vi "onDestroy.vi"(8 "error in (no error)":errorcluster, 11 "Client in":refnum<class "Client.lvclass">) -> (0 "error out":errorcluster, 3 "Client out":refnum<class "Client.lvclass">)   [LabVIEW 2013, in "MQTT Client.lvlib" / "Client.lvclass"]
uses:
  Client.lvclass
  MQTT_Base/Base Class/MQTT_Base.lvclass
  Client.lvclass/Client.ctl
  MQTT_Base/Session/Session.lvclass
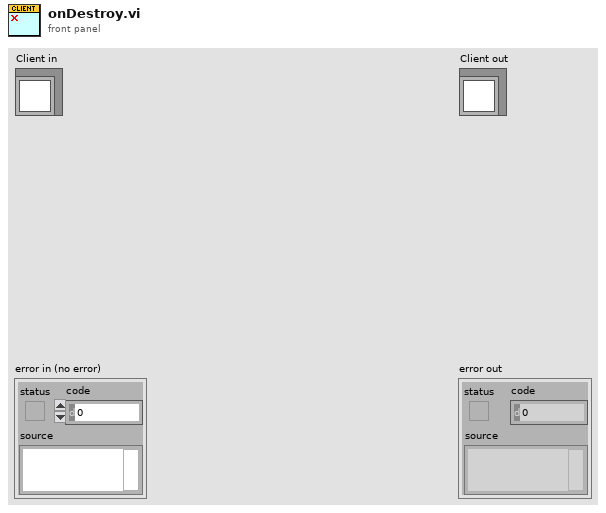
[diagram p1: front panel]
types:
  T1 = typedef "MQTT Client.lvlib/Client.lvclass/Public Events -- cluster.ctl" = cluster{"Connection Status":refnum<user-event>, "Connected":refnum<user-event>, "Application Message":refnum<user-event>}
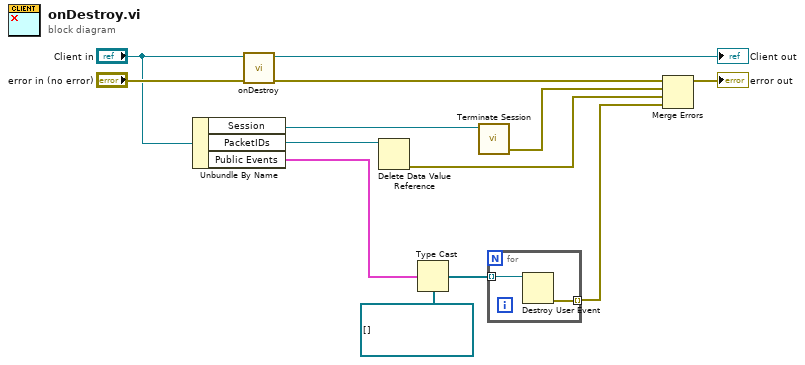
[diagram p0: block diagram]
diagram:
  n1 = Unbundle By Name("Client in") -> ("Session"=w9:refnum<class "Session.Client.lvclass">, "PacketIDs"=w10:refnum<data-value>, "Public Events"=w2:T1)
  n2 = call-parent "onDestroy.vi"("error in (no error)"="error in (no error)", "MQTT_Base in"="Client in") -> ("error out"=w8:errorcluster, "MQTT_Base out"=→"Client out":refnum<class "Client.lvclass">)  [unwired: 8 in]
  n3 = Delete Data Value Reference(data value reference=w10) -> (error out=w1:errorcluster)  [unwired: 1 in, 1 out]
  n4 = Type Cast(type=refnum<user-event>[] [], x=w2) -> (*(type *) &x=w4:refnum<user-event>[])
  n5 = call "Terminate Session.vi"("Session in"=w9) -> ("error out"=w6:errorcluster)  [unwired: 8 in, 2 out]
  n6 = for {
    tunnel: w4 -> [w15] mode=indexing
    tunnel: [w14] -> w3 mode=indexing
    n7 = Destroy User Event(user event=w15) -> (error out=w14:errorcluster)  [unwired: 1 in]
  }
  n8 = Merge Errors(w8, w6, w1, w3) -> (→"error out":errorcluster)
